vi "Get Server gRPC UEs.vi"(11 "OOP Server in":refnum<class "HVC7.lvclass">) -> (2 "Server gRPC UEs":T1, 3 "OOP Server out":refnum<class "HVC7.lvclass">)   [LabVIEW 2019, in "HVC7.lvlib" / "HVC7.lvclass"]
uses:
  HVC7.lvclass
  typeDefs/Server gRPC UEs.ctl
  gRPC lvSupport/Server API/typeDefs/gRPCId Cluster.ctl
  gRPC lvSupport/Server API/typeDefs/grpcId.ctl
  HVC7.lvclass/HVC7.ctl
  gRPC lvSupport/gprc-lvsupport.lvlib
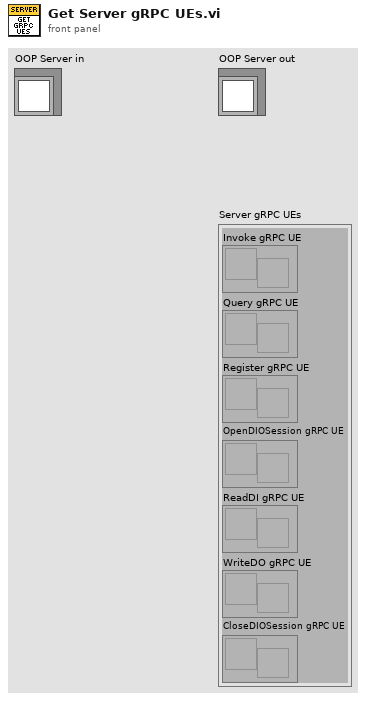
[diagram p1: front panel]
types:
  T1 = typedef "HVC7.lvlib/HVC7.lvclass/Server gRPC UEs.ctl" = cluster{"Invoke gRPC UE":refnum<user-event>, "Query gRPC UE":refnum<user-event>, "Register gRPC UE":refnum<user-event>, "OpenDIOSession gRPC UE":refnum<user-event>, "ReadDI gRPC UE":refnum<user-event>, "WriteDO gRPC UE":refnum<user-event>, "CloseDIOSession gRPC UE":refnum<user-event>}
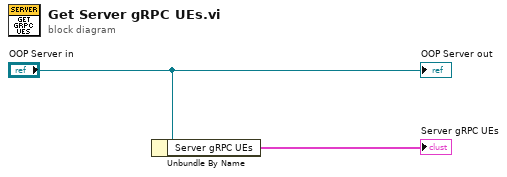
[diagram p0: block diagram]
diagram:
  n1 = Unbundle By Name("OOP Server in") -> ("Server gRPC UEs"=→"Server gRPC UEs":T1)
  "OOP Server out" <- "OOP Server in"
